vi "MyInterfaceMethod.vi"(0 "reference in":refnum<class "IMyInterface.lvclass">, 1 "MyParameter":dbl, 5 "error in (no error)":errorcluster) -> (14 "reference out":refnum<class "IMyInterface.lvclass">, 19 "error out":errorcluster)   [LabVIEW 2020, in "IMyInterface.lvclass"]
uses:
  IMyInterface.lvclass
  C:/Program Files (x86)/National Instruments/LabVIEW 2020/vi.lib/addons/_AddQ/G#Interface/G#Interface.lvclass
  <vilib>/addons/_AddQ/G#Interface/G#Interface.lvclass
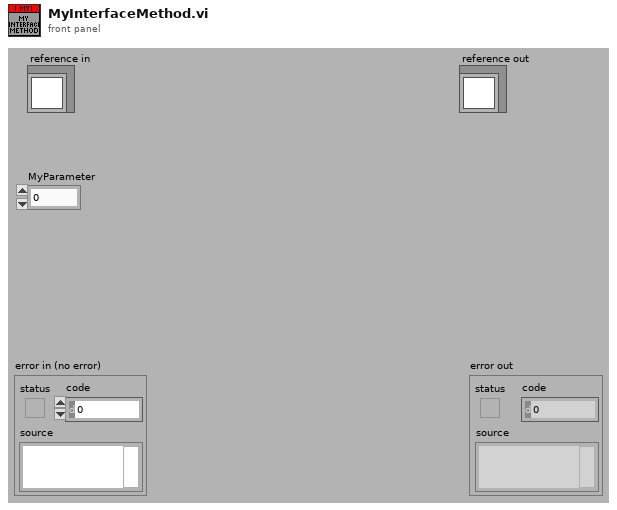
[diagram p1: front panel]
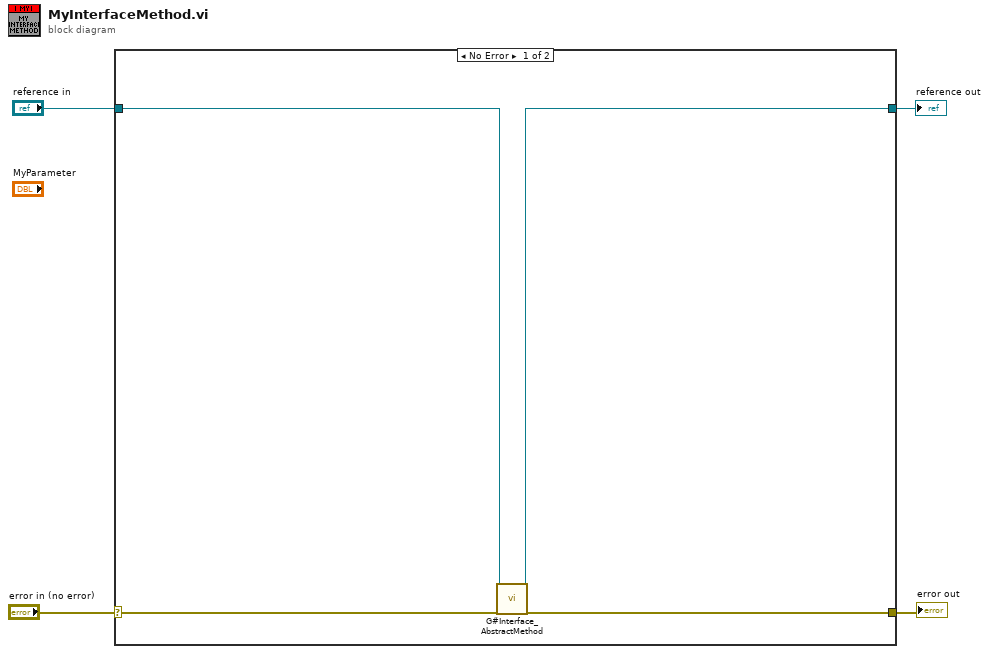
[diagram p0: block diagram]
diagram:
  n1 = case shown="No Error" "error in (no error)" {
    selector: "error in (no error)" -> [w7 w10]
    tunnel: [w8 w10] -> w3
    tunnel: [w5 w9] -> w1
    tunnel: "reference in" -> [w6 w9]
    frame No Error {
      n2 = call <vilib>:"G#Interface_AbstractMethod.vi"("reference in"=w6, "error in (no error)"=w7) -> ("reference out"=w5:refnum<class "IMyInterface.lvclass">, "error out"=w8:errorcluster)  [unwired: 16 in]
    }
    frame Error {
    }
  }
  "error out" <- w3
  "reference out" <- w1
